vi "1.vi"() -> ()   [LabVIEW 2013]
panel:
  in  "N":i32
  out "XY Graph":cluster{dbl[], dbl[]}(graph)
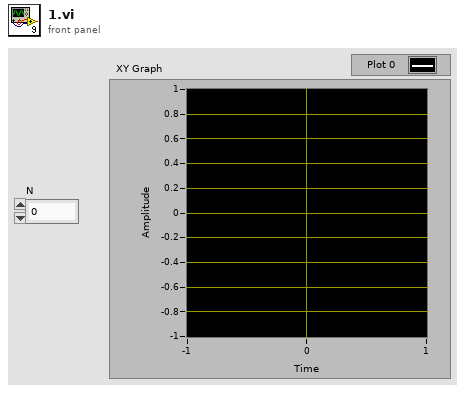
[diagram p1: front panel]
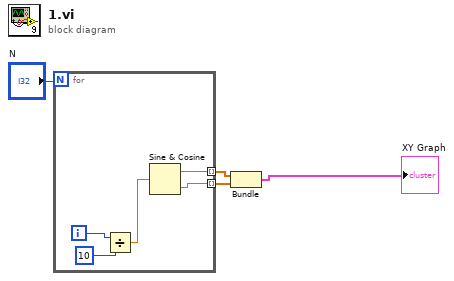
[diagram p0: block diagram]
diagram:
  n1 = for {
    N: "N" -> [_]
    tunnel: [w9] -> w4 mode=indexing
    tunnel: [w8] -> w3 mode=indexing
    i -> [w7]
    n2 = Divide(x=w7, y=10) -> (x/y=w5:dbl)
    n3 = Sine & Cosine(0:w5) -> (1:w9:dbl, 2:w8:dbl)
  }
  n4 = Bundle(w4, w3) -> (→"XY Graph":cluster{dbl[], dbl[]})  [unwired: 1 in]
